vi "LSM9DS1_RegGetSetRefNum.vi"(8 "error in (no error)":errorcluster, 9 "Operation":T3=enum."get", 10 "refnum name":string, 11 "LSM9DS1DevRef":T1={"DevStatus"={"status"=FALSE, "code"=0, "source"=""}, "Gyro Offset"={"Xzero"=0.0, "Yzero"=0.0, "Zzero"=0.0}, "StdDev Rates"={"Xsdo"=0.0, "Ysdo"=0.0, "Zsdo"=0.0}, "Reset"=FALSE, "Accel Offset"={"Xzero"=0.0, "Yzero"=0.0, "Zzero"=0.0}, "Motion Thresh"=0.0, "Mag Offset"={"Xzero"=1.0, "Yzero"=1.0, "Zzero"=1.0}, "I2C Bus"=enum."I2C On-Board", "Handle"=0, "Anomaly Thresh"=0.0, "Local Mag"=0.0, "Accel/Gyro_Address"=enum."0x6A", "Accel_Range"=enum."±2g", "Gyro_Range"=enum."±245dps", "Mag_Range"=enum."±2 gauss", "Mag_Address"=enum."0x1C", "accel_active"=FALSE, "gyro_active"=FALSE, "mag_active"=FALSE}) -> (0 "error out":errorcluster, 3 "LSM9DS1DevRef Out":T1={"DevStatus"={"status"=FALSE, "code"=0, "source"=""}, "Gyro Offset"={"Xzero"=0.0, "Yzero"=0.0, "Zzero"=0.0}, "StdDev Rates"={"Xsdo"=0.0, "Ysdo"=0.0, "Zsdo"=0.0}, "Reset"=FALSE, "Accel Offset"={"Xzero"=0.0, "Yzero"=0.0, "Zzero"=0.0}, "Motion Thresh"=0.0, "Mag Offset"={"Xzero"=1.0, "Yzero"=1.0, "Zzero"=1.0}, "I2C Bus"=enum."I2C On-Board", "Handle"=0, "Anomaly Thresh"=0.0, "Local Mag"=0.0, "Accel/Gyro_Address"=enum."0x6A", "Accel_Range"=enum."±2g", "Gyro_Range"=enum."±245dps", "Mag_Range"=enum."±2 gauss", "Mag_Address"=enum."0x1C", "accel_active"=FALSE, "gyro_active"=FALSE, "mag_active"=FALSE})   [LabVIEW 2015]
doc: "Sets a reference into a registry, gets a reference from a registry, or deletes a reference from a registry. The reference is accessed by name, and can be given any unique name.\n\nThis software is licensed. Open the labview\\readme\\WPI Robotics Library Open Source License.txt file for more information."
uses:
  <vilib>/Rock Robotics/WPI/Utilities/Refnum Registry Operation.ctl
  LSM9DS1DevRef.ctl
  <vilib>/Rock Robotics/SystemInterfaces/i2clib/i2c_bus.ctl
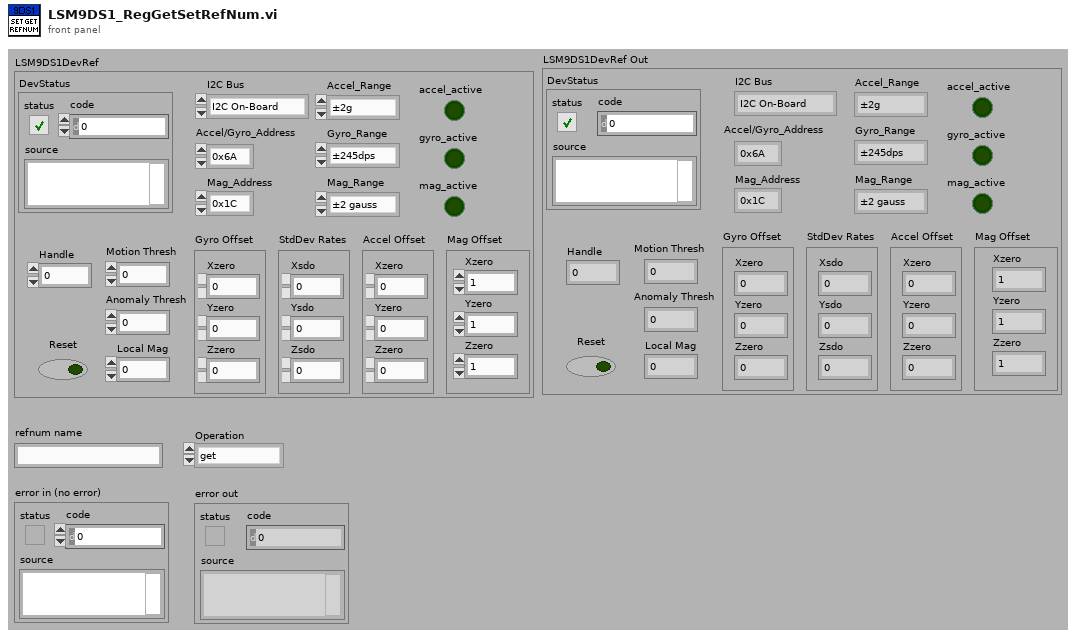
[diagram p1: front panel]
types:
  T1 = typedef "LSM9DS1DevRef.ctl" = cluster{"DevStatus":errorcluster, "Gyro Offset":cluster{"Xzero":dbl, "Yzero":dbl, "Zzero":dbl}, "StdDev Rates":cluster{"Xsdo":dbl, "Ysdo":dbl, "Zsdo":dbl}, "Reset":bool, "Accel Offset":cluster{"Xzero":dbl, "Yzero":dbl, "Zzero":dbl}, "Motion Thresh":dbl, "Mag Offset":cluster{"Xzero":dbl, "Yzero":dbl, "Zzero":dbl}, "I2C Bus":T2, "Handle":i32, "Anomaly Thresh":dbl, "Local Mag":dbl, "Accel/Gyro_Address":enum8{"0x6A", "0x6B"}, "Accel_Range":enum16{"±2g", "±16g", "±4g", "±8g", "disabled"}, "Gyro_Range":enum16{"±245dps", "±500dps", "disabled", "±2000dps"}, "Mag_Range":enum16{"±2 gauss", "±4 gauss", "±8 gauss", "±16 gauss", "disabled"}, "Mag_Address":enum8{"0x1C", "0x1E"}, "accel_active":bool, "gyro_active":bool, "mag_active":bool}
  T2 = typedef "i2c_bus.ctl" = enum16{"I2C On-Board", "I2C MXP", "Invalid"}
  T3 = typedef "Refnum Registry Operation.ctl" = enum16{"set", "get", "delete", "get all names", "read name"}
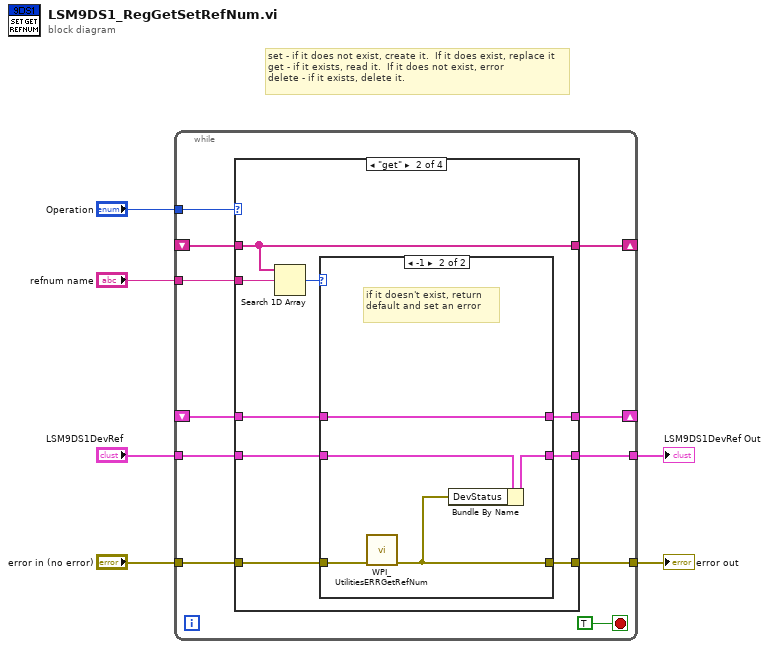
[diagram p0: block diagram]
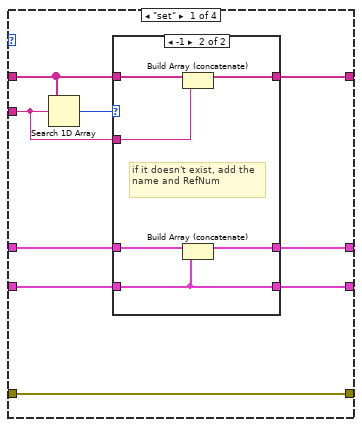
[diagram p2: hidden frame]
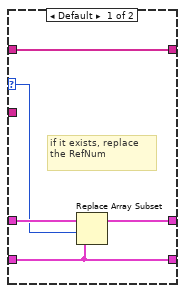
[diagram p3: hidden frame]
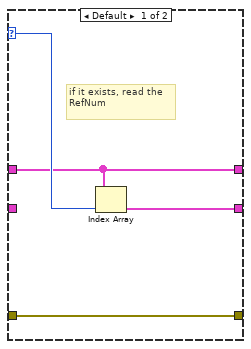
[diagram p4: hidden frame]
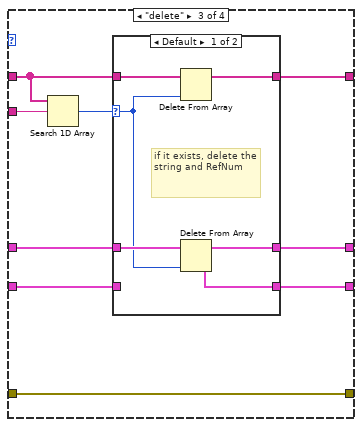
[diagram p5: hidden frame]
diagram:
  # "set - if it does not exist, create it.  If it does exist, replace it\nget - if it exists, read it.  If it does not exist, error\ndelete - if it exists, delete it."
  n1 = while {
    tunnel: "LSM9DS1DevRef" -> [w17]
    tunnel: "refnum name" -> [w10]
    tunnel: "error in (no error)" -> [w9]
    shift-right: [w16] -> _
    shift-left: _ -> [w15]
    tunnel: [w14] -> w1
    tunnel: "Operation" -> [w13]
    shift-right: [w12] -> _
    shift-left: _ -> [w11]
    tunnel: [w8] -> w4
    stop <- TRUE stop-if-true
    n2 = case shown="\"get\"" w13 {
      tunnel: w17 -> [w21 w43 w59 w76]
      tunnel: [w20 w42 w58 w77] -> w16
      tunnel: w15 -> [w22 w44 w60 w77]
      tunnel: [w19 w41 w57 w76] -> w14
      tunnel: [w26 w40 w64 w74] -> w12
      tunnel: w11 -> [w25 w40 w63 w74]
      tunnel: w10 -> [w23 w45 w61 _]
      tunnel: [w18 w38 w56 w75] -> w8
      tunnel: w9 -> [w18 w39 w56 w75]
      frame "set" {
        n3 = Search 1D Array(1D array=w25, element=w23) -> (index of element=w24:i32)  [unwired: 1 out]
        n4 = case shown="-1" w24 {
          selector: w24 -> [w29 _]
          tunnel: [w31 w37] -> w26
          tunnel: w25 -> [w31 w36]
          tunnel: w23 -> [_ w35]
          tunnel: w22 -> [w30 w34]
          tunnel: w21 -> [w27 w32]
          tunnel: [w28 w33] -> w20
          tunnel: [w27 w32] -> w19
          frame Default {
            # "if it exists, replace the RefNum"
            n5 = Replace Array Subset(array=w30, new element=w27, index=w29) -> (w28:T1[])
          }
          frame -1 {
            # "if it doesn't exist, add the name and RefNum"
            n6 = Build Array (concatenate)(w36, w35) -> (w37:string[])
            n7 = Build Array (concatenate)(w34, w32) -> (w33:T1[])
          }
        }
      }
      frame "get" {
        n8 = Search 1D Array(1D array=w40, element=w45) -> (index of element=w46:i32)  [unwired: 1 out]
        n9 = case shown="-1" w46 {
          selector: w46 -> [w50 _]
          tunnel: w44 -> [w48 w55]
          tunnel: w43 -> [_ w53]
          tunnel: [w48 w55] -> w42
          tunnel: [w49 w52] -> w41
          tunnel: w39 -> [w47 w54]
          tunnel: [w47 w51] -> w38
          frame Default {
            # "if it exists, read the RefNum"
            n10 = Index Array(array=w48, index=w50) -> (element=w49:T1)
          }
          frame -1 {
            # "if it doesn't exist, return default and set an error"
            n11 = call <vilib>:"WPI_UtilitiesERRGetRefNum.vi"("error in (no error)"=w54) -> ("ERRGetRefNum"=w51:errorcluster)  [unwired: 10 out]
            n12 = Bundle By Name(cluster=w53, "DevStatus"=w51) -> (w52:T1)
          }
        }
      }
      frame "delete" {
        n13 = Search 1D Array(1D array=w63, element=w61) -> (index of element=w62:i32)  [unwired: 1 out]
        n14 = case shown="Default" w62 {
          selector: w62 -> [w65 _]
          tunnel: [w66 w72] -> w64
          tunnel: w63 -> [w67 w72]
          tunnel: w60 -> [w70 w71]
          tunnel: w59 -> [_ w73]
          tunnel: [w69 w71] -> w58
          tunnel: [w68 w73] -> w57
          frame Default {
            # "if it exists, delete the string and RefNum"
            n15 = Delete From Array(array=w67, index=w65) -> (array with subset deleted=w66:string[])  [unwired: 1 in, 1 out]
            n16 = Delete From Array(array=w70, index=w65) -> (deleted portion=w68:T1, array with subset deleted=w69:T1[])  [unwired: 1 in]
          }
          frame -1 {
            # "if it doesn't exist, do nothing"
          }
        }
      }
      frame "get all names", Default {
      }
    }
  }
  "error out" <- w4
  "LSM9DS1DevRef Out" <- w1
